vi "Signals.vi"() -> ()   [LabVIEW 2019]
uses:
  <vilib>/Analysis/NI_AALBase.lvlib
panel:
  in  "stop":bool
  out "Waveform Chart":dynamicdata(graph)
  in  "Frequency":dbl(knob) scale=0.0..10.0
  in  "Amplitude":dbl(knob) scale=0.0..10.0
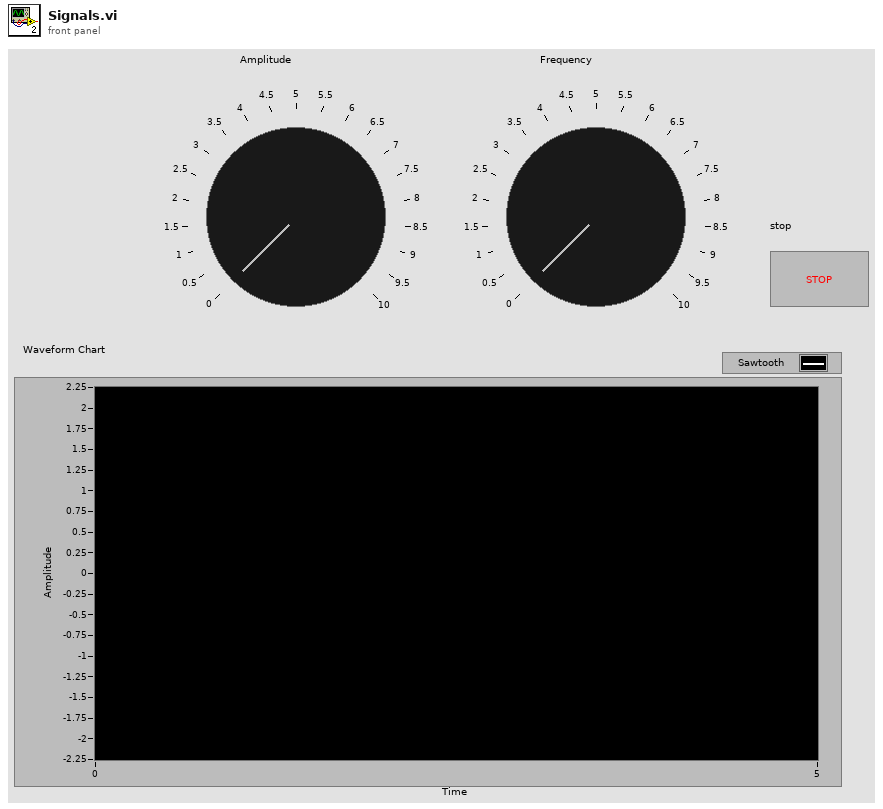
[diagram p1: front panel]
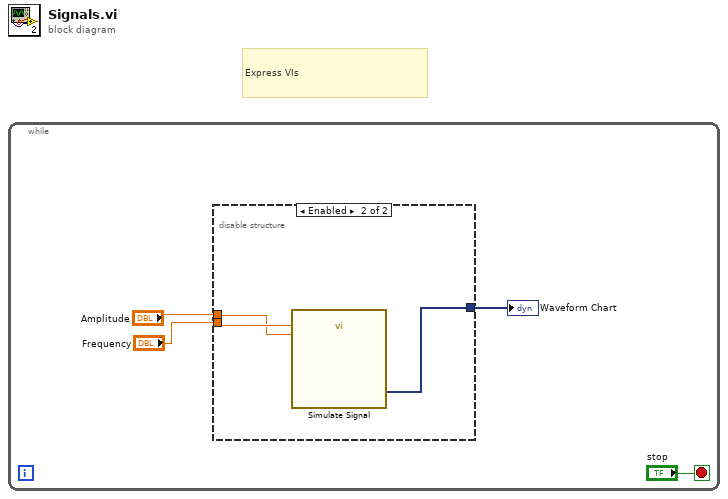
[diagram p0: block diagram]
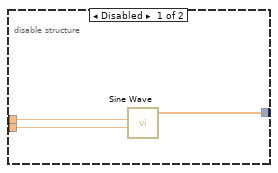
[diagram p2: hidden frame]
diagram:
  # "Express VIs"
  n1 = while {
    stop <- "stop" stop-if-true
    n2 = disable-structure shown="Enabled" {
      disable-tunnel: "Amplitude" -> [w7 w9]
      disable-tunnel: "Frequency" -> [w6 w10]
      disable-tunnel: [w5 w8] -> w2
      frame Disabled {
        n3 = call <vilib>:"Sine Wave.vi"("amplitude"=w7, "frequency"=w6) -> ("sine wave"=w5:dbl[])  [unwired: 3 in, 2 out]
      }
      frame Enabled {
        n4 = call "Simulate Signal"("Frequency"=w10, "Amplitude"=w9) -> ("Sawtooth"=w8:dynamicdata)  [unwired: 12 in, 1 out]
      }
    }
    "Waveform Chart" <- w2
  }
